vi "PBC_Telemetry.vi"(10 "Variant":variant) -> (2 "Telemetry":T1 {"Raw_Telemetry" format="%04x"; "Register 0"."PBC_Rev" format="%02x"; "Register 0"."PBC_Fuse" format="%02x"; "Register 0"."PBC_ID" format="%02x"; "Register 1"."VSA_CPT[3:1]" format="%02x"; "Register 2"."Saltaper" format="%01x"; "Register 3"."WDOG_Count" format="%04x"; "Register 3"."CRD_BDDR" format="%02x"; "Register 6"."cntValCMD_A[15:8]" format="%02x"; "Register 6"."cntBadCMD_A[7:0]" format="%02x"; "Register 7"."cntValCMD_B[15:8]" format="%02x"; "Register 7"."cntBadCMD_B[7:0]" format="%02x"; "Register 8"."Ki" format="%04x"; "Register 9"."Kp" format="%04x"; "Register 10"."Kd" format="%04x"; "Register 11"."VoltTapSp" format="%02x"; "Register 11"."CurrSp" format="%02x"; "Register 11"."voltSp" format="%02x"; "Register 12"."Reserved" format="%02x"; "Register 12"."IV_DAC" format="%04x"; "Register 15"."Vcps" format="%04x"; "Register 16"."AH_I_MSW" format="%04x"; "Register 17"."AH_I_LSW" format="%04x"; "Register 18"."Curr_Sp" format="%04x"; "Register 19"."DEBUG" format="%04x"})   [LabVIEW 2019, in "Variant Parser.lvlib" / "Variant Parser.lvclass"]
uses:
  Library/Variant Parser.lvclass
panel:
  # "Volt Taper Setpoint"
  # "Current Setpoint"
  # "Volt Setpoint"
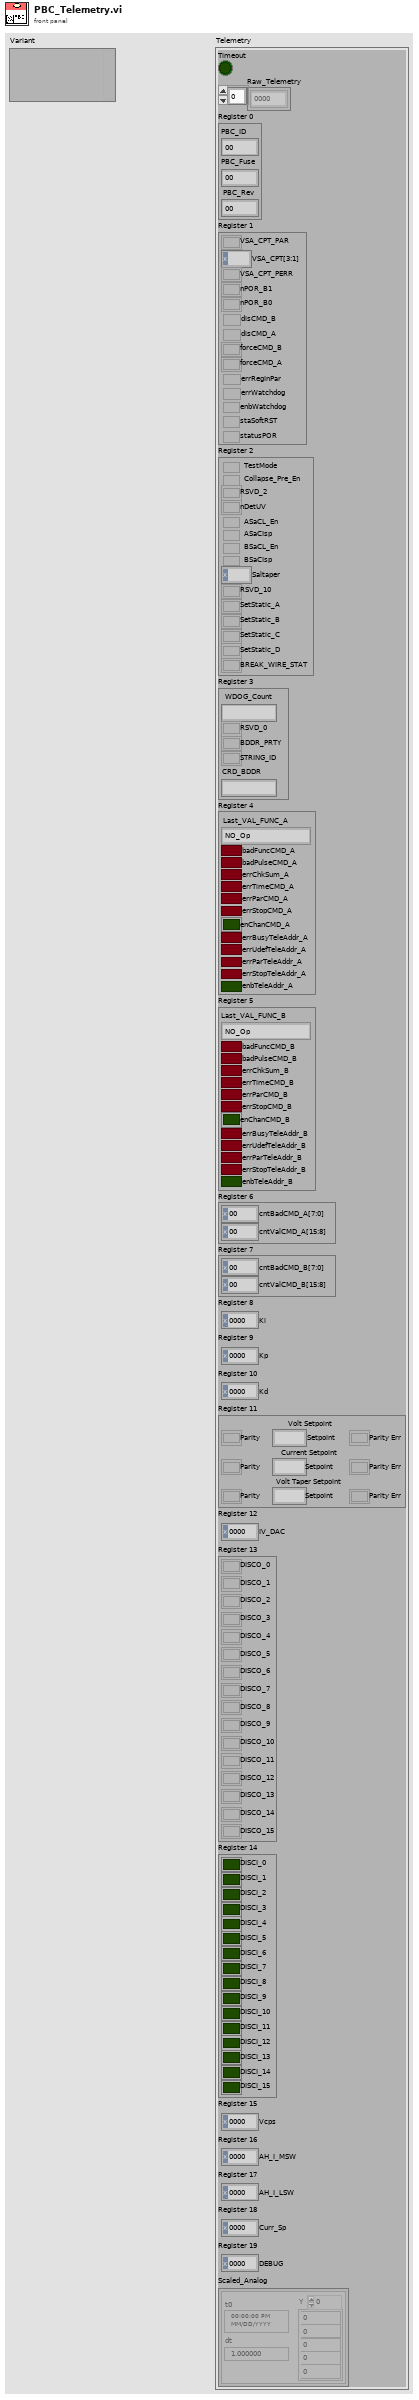
[diagram p1: front panel]
types:
  T1 = cluster{"Timeout":bool, "Raw_Telemetry":u16[], "Register 0":cluster{"PBC_ID":u8, "PBC_Fuse":u8, "PBC_Rev":u8}, "Register 1":cluster{"VSA_CPT_PAR":bool, "VSA_CPT[3:1]":u8, "VSA_CPT_PERR":bool, "nPOR_B1":bool, "nPOR_B0":bool, "disCMD_B":bool, "disCMD_A":bool, "forceCMD_B":bool, "forceCMD_A":bool, "errRegInPar":bool, "errWatchdog":bool, "enbWatchdog":bool, "staSoftRST":bool, "statusPOR":bool}, "Register 2":cluster{"TestMode":bool, "Collapse_Pre_En":bool, "RSVD_2":bool, "nDetUV":bool, "ASaCL_En":bool, "ASaCIsp":bool, "BSaCL_En":bool, "BSaCIsp":bool, "Saltaper":u8, "RSVD_10":bool, "SetStatic_A":bool, "SetStatic_B":bool, "SetStatic_C":bool, "SetStatic_D":bool, "BREAK_WIRE_STAT":bool}, "Register 3":cluster{"CRD_BDDR":u8, "STRING_ID":bool, "BDDR_PRTY":bool, "RSVD_0":bool, "WDOG_Count":u16}, "Register 4":cluster{"Last_VAL_FUNC_A":enum16{"NO_Op", "Static_Discrete", "Housekeeping", "Memory_Command", "Bad_Command"}, "badFuncCMD_A":bool, "badPulseCMD_A":bool, "errChkSum_A":bool, "errTimeCMD_A":bool, "errParCMD_A":bool, "errStopCMD_A":bool, "enChanCMD_A":bool, "errBusyTeleAddr_A":bool, "errUdefTeleAddr_A":bool, "errParTeleAddr_A":bool, "errStopTeleAddr_A":bool, "enbTeleAddr_A":bool}, "Register 5":cluster{"Last_VAL_FUNC_B":enum16{"NO_Op", "Static_Discrete", "Housekeeping", "Memory_Command", "Bad_Command"}, "badFuncCMD_B":bool, "badPulseCMD_B":bool, "errChkSum_B":bool, "errTimeCMD_B":bool, "errParCMD_B":bool, "errStopCMD_B":bool, "enChanCMD_B":bool, "errBusyTeleAddr_B":bool, "errUdefTeleAddr_B":bool, "errParTeleAddr_B":bool, "errStopTeleAddr_B":bool, "enbTeleAddr_B":bool}, "Register 6":cluster{"cntBadCMD_A[7:0]":u8, "cntValCMD_A[15:8]":u8}, "Register 7":cluster{"cntBadCMD_B[7:0]":u8, "cntValCMD_B[15:8]":u8}, "Register 8":cluster{"Ki":u16}, "Register 9":cluster{"Kp":u16}, "Register 10":cluster{"Kd":u16}, "Register 11":cluster{"voltSpPar":bool, "voltSp":u8, "voltSpParErr":bool, "CurrSpParErr":bool, "CurrSp":u8, "CurrSpPar":bool, "VoltTapSpParErr":bool, "VoltTapSp":u8, "VoltTapPar":bool}, "Register 12":cluster{"IV_DAC":u16, "Reserved":u8}, "Register 13":cluster{"DISCO_0":bool, "DISCO_1":bool, "DISCO_2":bool, "DISCO_3":bool, "DISCO_4":bool, "DISCO_5":bool, "DISCO_6":bool, "DISCO_7":bool, "DISCO_8":bool, "DISCO_9":bool, "DISCO_10":bool, "DISCO_11":bool, "DISCO_12":bool, "DISCO_13":bool, "DISCO_14":bool, "DISCO_15":bool}, "Register 14":cluster{"DISCI_0":bool, "DISCI_1":bool, "DISCI_2":bool, "DISCI_3":bool, "DISCI_4":bool, "DISCI_5":bool, "DISCI_6":bool, "DISCI_7":bool, "DISCI_8":bool, "DISCI_9":bool, "DISCI_10":bool, "DISCI_11":bool, "DISCI_12":bool, "DISCI_13":bool, "DISCI_14":bool, "DISCI_15":bool}, "Register 15":cluster{"Vcps":u16}, "Register 16":cluster{"AH_I_MSW":u16}, "Register 17":cluster{"AH_I_LSW":u16}, "Register 18":cluster{"Curr_Sp":u16}, "Register 19":cluster{"DEBUG":u16}, "Scaled_Analog":waveform(dbl)[]}
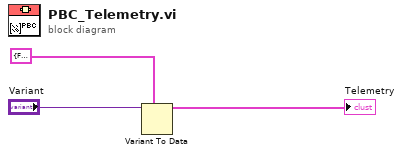
[diagram p0: block diagram]
diagram:
  n1 = Variant To Data(type=T1 {"Timeout"=FALSE, "Raw_Telemetry"=[], "Register 0"={"PBC_ID"=0, "PBC_Fuse"=0, "PBC_Rev"=0}, "Register 1"={"VSA_CPT_PAR"=FALSE, "VSA_CPT[3:1]"=0, "VSA_CPT_PERR"=FALSE, "nPOR_B1"=FALSE, "nPOR_B0"=FALSE, "disCMD_B"=FALSE, "disCMD_A"=FALSE, "forceCMD_B"=FALSE, "forceCMD_A"=FALSE, "errRegInPar"=FALSE, "errWatchdog"=FALSE, "enbWatchdog"=FALSE, "staSoftRST"=FALSE, "statusPOR"=FALSE}, "Register 2"={"TestMode"=FALSE, "Collapse_Pre_En"=FALSE, "RSVD_2"=FALSE, "nDetUV"=FALSE, "ASaCL_En"=FALSE, "ASaCIsp"=FALSE, "BSaCL_En"=FALSE, "BSaCIsp"=FALSE, "Saltaper"=0, "RSVD_10"=FALSE, "SetStatic_A"=FALSE, "SetStatic_B"=FALSE, "SetStatic_C"=FALSE, "SetStatic_D"=FALSE, "BREAK_WIRE_STAT"=FALSE}, "Register 3"={"CRD_BDDR"=0, "STRING_ID"=FALSE, "BDDR_PRTY"=FALSE, "RSVD_0"=FALSE, "WDOG_Count"=0}, "Register 4"={"Last_VAL_FUNC_A"=enum."NO_Op", "badFuncCMD_A"=FALSE, "badPulseCMD_A"=FALSE, "errChkSum_A"=FALSE, "errTimeCMD_A"=FALSE, "errParCMD_A"=FALSE, "errStopCMD_A"=FALSE, "enChanCMD_A"=FALSE, "errBusyTeleAddr_A"=FALSE, "errUdefTeleAddr_A"=FALSE, "errParTeleAddr_A"=FALSE, "errStopTeleAddr_A"=FALSE, "enbTeleAddr_A"=FALSE}, "Register 5"={"Last_VAL_FUNC_B"=enum."NO_Op", "badFuncCMD_B"=FALSE, "badPulseCMD_B"=FALSE, "errChkSum_B"=FALSE, "errTimeCMD_B"=FALSE, "errParCMD_B"=FALSE, "errStopCMD_B"=FALSE, "enChanCMD_B"=FALSE, "errBusyTeleAddr_B"=FALSE, "errUdefTeleAddr_B"=FALSE, "errParTeleAddr_B"=FALSE, "errStopTeleAddr_B"=FALSE, "enbTeleAddr_B"=FALSE}, "Register 6"={"cntBadCMD_A[7:0]"=0, "cntValCMD_A[15:8]"=0}, "Register 7"={"cntBadCMD_B[7:0]"=0, "cntValCMD_B[15:8]"=0}, "Register 8"={"Ki"=0}, "Register 9"={"Kp"=0}, "Register 10"={"Kd"=0}, "Register 11"={"voltSpPar"=FALSE, "voltSp"=0, "voltSpParErr"=FALSE, "CurrSpParErr"=FALSE, "CurrSp"=0, "CurrSpPar"=FALSE, "VoltTapSpParErr"=FALSE, "VoltTapSp"=0, "VoltTapPar"=FALSE}, "Register 12"={"IV_DAC"=0, "Reserved"=0}, "Register 13"={"DISCO_0"=FALSE, "DISCO_1"=FALSE, "DISCO_2"=FALSE, "DISCO_3"=FALSE, "DISCO_4"=FALSE, "DISCO_5"=FALSE, "DISCO_6"=FALSE, "DISCO_7"=FALSE, "DISCO_8"=FALSE, "DISCO_9"=FALSE, "DISCO_10"=FALSE, "DISCO_11"=FALSE, "DISCO_12"=FALSE, "DISCO_13"=FALSE, "DISCO_14"=FALSE, "DISCO_15"=FALSE}, "Register 14"={"DISCI_0"=FALSE, "DISCI_1"=FALSE, "DISCI_2"=FALSE, "DISCI_3"=FALSE, "DISCI_4"=FALSE, "DISCI_5"=FALSE, "DISCI_6"=FALSE, "DISCI_7"=FALSE, "DISCI_8"=FALSE, "DISCI_9"=FALSE, "DISCI_10"=FALSE, "DISCI_11"=FALSE, "DISCI_12"=FALSE, "DISCI_13"=FALSE, "DISCI_14"=FALSE, "DISCI_15"=FALSE}, "Register 15"={"Vcps"=0}, "Register 16"={"AH_I_MSW"=0}, "Register 17"={"AH_I_LSW"=0}, "Register 18"={"Curr_Sp"=0}, "Register 19"={"DEBUG"=0}, "Scaled_Analog"=[]}, Variant="Variant") -> (data=→"Telemetry":T1)  [unwired: 1 in, 1 out]
